vi "Server.vi"() -> ()   [LabVIEW 2016]
uses:
  C:/Users/Administrator/Desktop/HslCommunicationDemo-v5.7.0/HslCommunication.dll
  HslCommunication.dll
panel:
  out "OnlineCount":i32
  out "推送随机数":string
  in  "停止按钮":bool
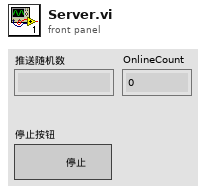
[diagram p1: front panel]
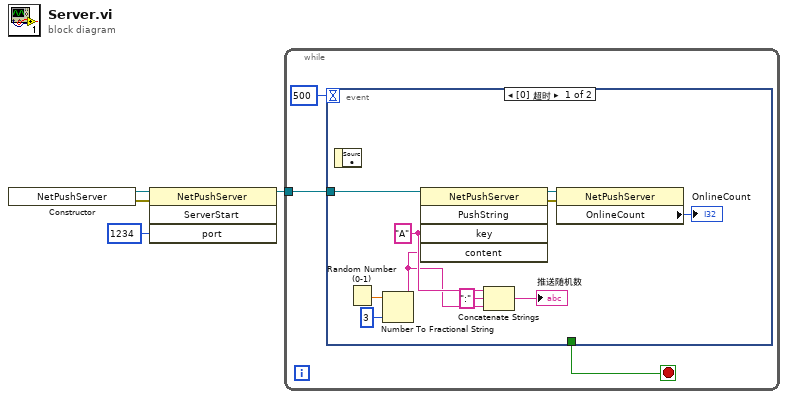
[diagram p0: block diagram]
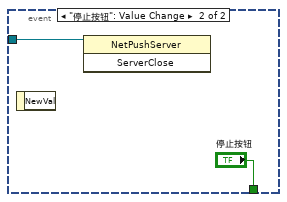
[diagram p2: hidden frame]
diagram:
  n1 = constructor class="NetPushServer"() -> (reference out=w3:refnum<k24>, error out=w4:errorcluster)  [unwired: 3 in, 1 out]
  n2 = invoke class="NetPushServer" method="ServerStart"(reference=w3, error in=w4, "port"=1234) -> (reference out=w1:refnum<k24>)  [unwired: 1 in, 3 out]
  n3 = while {
    tunnel: w1 -> [w5]
    stop <- w7 stop-if-true
    n4 = event shown="[0] 超时" {
      selector: _ -> [_ _]
      dyn-events: _ -> [_ _]
      timeout: 500 -> [_ _]
      tunnel: [_ "停止按钮"] -> w7
      tunnel: w5 -> [w17 w18]
      event Timeout {
        w14 = "A" ("key")
        n5 = event-data() -> ()  [unwired: 1 in, 1 out]
        n6 = Random Number (0-1)() -> (number: 0 to 1=w16:dbl)
        n7 = Number To Fractional String(number=w16, precision (6)=i16 3 ("精度(6)")) -> (F-format string=w12:string)  [unwired: 2 in]
        n8 = invoke class="NetPushServer" method="PushString"(reference=w17, "key"=w14, "content"=w12) -> (reference out=w9:refnum<k24>, error out=w10:errorcluster)  [unwired: 2 in, 3 out]
        n9 = Concatenate Strings(w14, ":" ("字符串"), w12) -> (→"推送随机数":string)
        n10 = property class="NetPushServer"(reference=w9, error in=w10) -> ("OnlineCount"=→"OnlineCount":i32)  [unwired: 2 out]
      }
      event "停止按钮": Value Change {
        n11 = event-data() -> ()  [unwired: 1 in, 1 out]
        n12 = invoke class="NetPushServer" method="ServerClose"(reference=w18) -> ()  [unwired: 2 in, 3 out]
      }
    }
  }
